vi "4 BIT Register.vi"(1 "Clock":bool, 2 "Data In":bool[](array[boolean])=[FALSE, FALSE, FALSE, FALSE, FALSE, FALSE, FALSE, FALSE, FALSE, FALSE, FALSE, FALSE, FALSE, FALSE, FALSE, FALSE], 3 "Hold":bool) -> (0 "Data Out":bool[](array[boolean]))   [LabVIEW 2012]
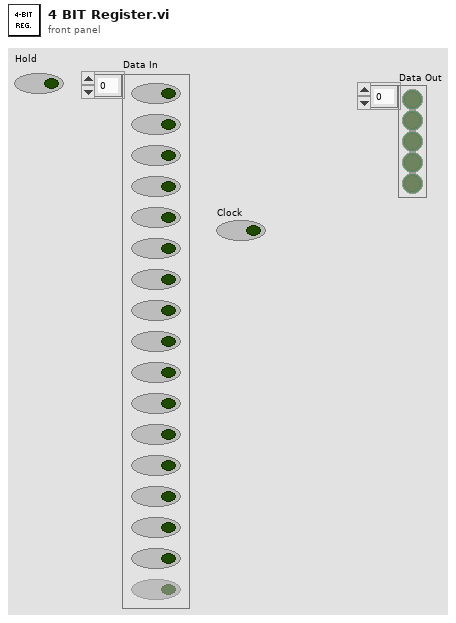
[diagram p1: front panel]
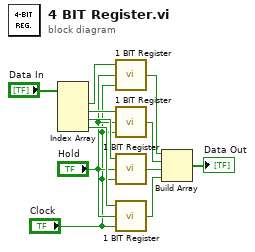
[diagram p0: block diagram]
diagram:
  n1 = Index Array(array="Data In") -> (element #1=w11:bool, element #2=w10:bool, element #3=w9:bool, element #4=w8:bool)  [unwired: 4 in]
  n2 = call "1 BIT Register.vi"("Clock"="Clock", "Hold"="Hold", "Data"=w11) -> ("Q"=w6:bool)
  n3 = call "1 BIT Register.vi"("Clock"="Clock", "Hold"="Hold", "Data"=w10) -> ("Q"=w5:bool)
  n4 = call "1 BIT Register.vi"("Clock"="Clock", "Hold"="Hold", "Data"=w9) -> ("Q"=w4:bool)
  n5 = call "1 BIT Register.vi"("Clock"="Clock", "Hold"="Hold", "Data"=w8) -> ("Q"=w3:bool)
  n6 = Build Array(w6, w5, w4, w3) -> (→"Data Out":bool[])
